vi "PathFinder.vi"() -> (1 "Save?":bool, 3 "selected path":path)   [LabVIEW 2012, in "Data Logger.lvlib" / "Data Logger.lvclass"]
uses:
  Data Logger.lvclass
  PathFinder Type def.ctl
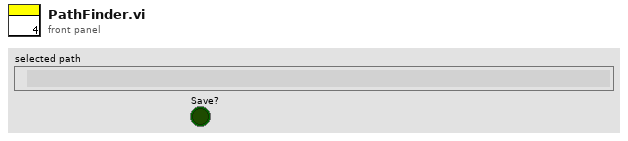
[diagram p1: front panel]
types:
  T1 = typedef "PathFinder Type def.ctl" = enum16{"Done", "Waiting"}
  T2 = cluster{"Project Number":string, "Manufacturer":string, "Model":string, "Serial":string, "Comment":string}
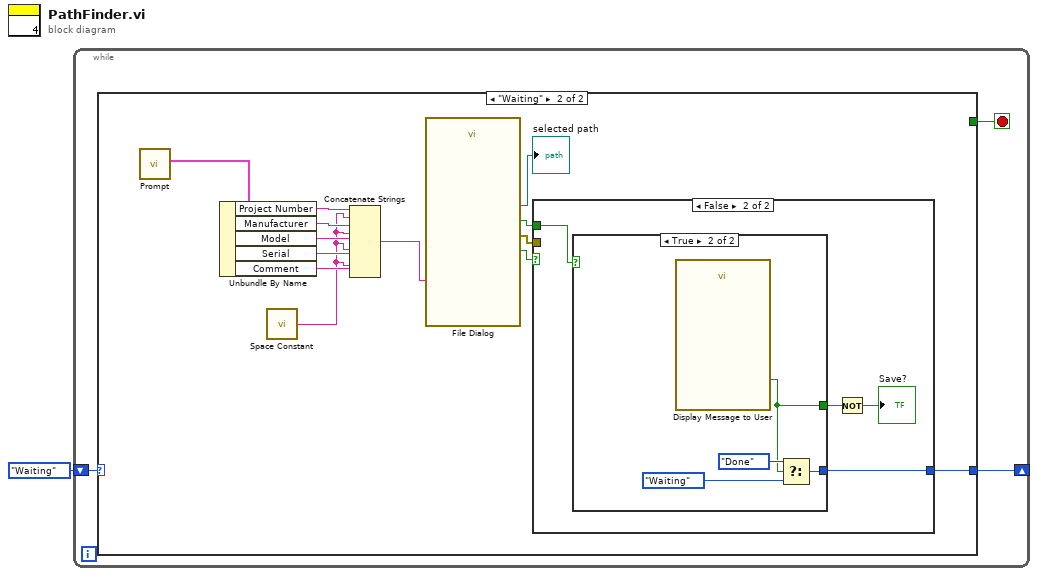
[diagram p0: block diagram]
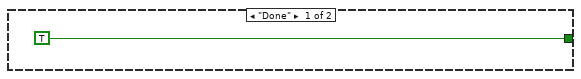
[diagram p2: hidden frame]
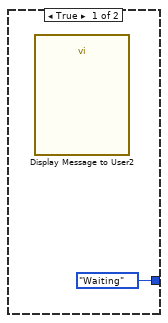
[diagram p3: hidden frame]
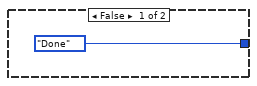
[diagram p4: hidden frame]
diagram:
  n1 = while {
    shift-right: [w2] -> _
    shift-left: PathFinder_Type_def."Waiting" -> [w4]
    stop <- w3 stop-if-true
    n2 = case shown="\"Waiting\"" w4 {
      tunnel: [TRUE _] -> w3
      tunnel: [_ w16] -> w2
      frame "Done" {
      }
      frame "Waiting" {
        n3 = call "Prompt.vi"() -> ("Cluster"=w13:T2)  [unwired: 11 in]
        n4 = Unbundle By Name(w13) -> ("Project Number"=w12:string, "Manufacturer"=w11:string, "Model"=w10:string, "Serial"=w9:string, "Comment"=w8:string)
        n5 = call <vilib>:"Space Constant.vi"() -> ("String"=w7:string)
        n6 = Concatenate Strings(w12, w7, w11, w7, w10, w7, w9, w7, w8) -> (w6:string)
        n7 = call "File Dialog"("default name"=w6) -> ("selected path"=→"selected path":path, "exists"=w17:bool, "cancelled"=w18:bool, "error out"=w15:errorcluster)  [unwired: 11 in]
        n8 = case shown="False" w17 {
          tunnel: w18 -> [_ w23]
          tunnel: [PathFinder_Type_def."Waiting" w22] -> w16
          tunnel: w15 -> [_ _]
          frame True {
            n9 = call "Display Message to User2"() -> ()  [unwired: 10 in, 2 out]
          }
          frame False {
            n10 = case shown="True" w23 {
              tunnel: [PathFinder_Type_def."Done" w26] -> w22
              tunnel: [_ w25] -> w21
              frame False {
              }
              frame True {
                n11 = call "Display Message to User"() -> ("Do Not Save"=w25:bool)  [unwired: 10 in, 1 out]
                n12 = Select(t=PathFinder_Type_def."Done", s=w25, f=PathFinder_Type_def."Waiting") -> (s? t:f=w26:T1)
              }
            }
            n13 = Not(x=w21) -> (.not. x?=→"Save?":bool)
          }
        }
      }
    }
  }
